vi "central difference.vi"   [LabVIEW 2010, in "common.lvlib"]
uses:
  common.lvlib
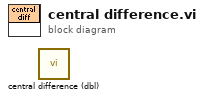
[diagram p0: block diagram]
diagram:
  n1 = call "central difference (dbl).vi"() -> ()  [unwired: 5 in, 1 out]
